vi "test ClearData.vi"(8 "error in (no error)":errorcluster, 11 "TestCase in":refnum<class "Data Manipulation Tests.lvclass">) -> (0 "error out":errorcluster, 3 "TestCase out":refnum<class "Data Manipulation Tests.lvclass">)   [LabVIEW 2017, in "Pointer Tests.lvlib" / "Data Manipulation Tests.lvclass"]
uses:
  Data Manipulation Tests.lvclass
  Source/Classes/Pointer/Public/New/New (1B).vi
  Source/Classes/Pointer/Public/Write/Write (1D U8).vi
  Source/Classes/Pointer/Public/Read/Read (1D U8).vi
  <vilib>/addons/_JKI Toolkits/VI Tester/TestCase.llb/TestCase.lvclass
  Source/Classes/Pointer/Pointer.lvclass
  C:/Program Files (x86)/National Instruments/LabVIEW 2017/vi.lib/addons/_JKI Toolkits/VI Tester/TestCase.llb/TestCase.lvclass
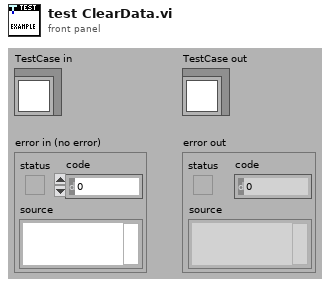
[diagram p1: front panel]
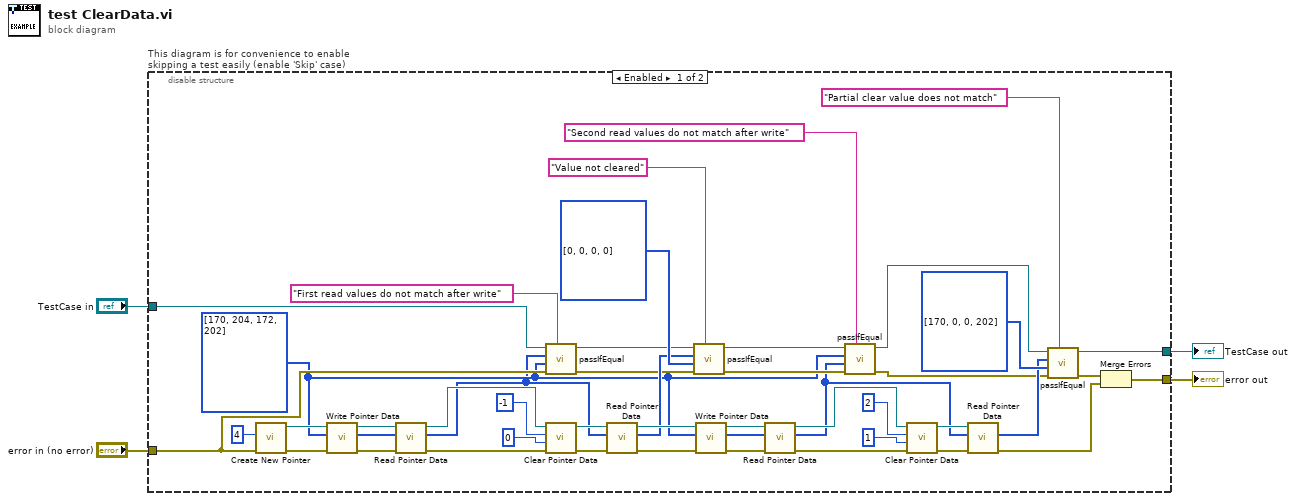
[diagram p0: block diagram]
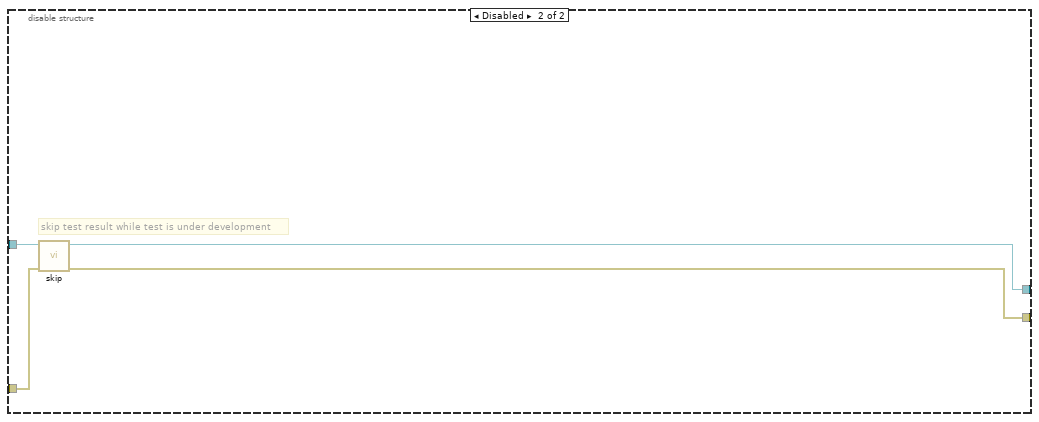
[diagram p2: hidden frame]
diagram:
  n1 = disable-structure "This diagram is for convenience to enable skipping a test easily (enable 'Skip' case)" shown="Enabled" {
    disable-tunnel: "TestCase in" -> [w23 w54]
    disable-tunnel: [w41 w52] -> w1
    disable-tunnel: [w38 w53] -> w3
    disable-tunnel: "error in (no error)" -> [w21 w51]
    frame Enabled {
      w9 = u8[] [170, 204, 172, 202] ("buffer in")
      n2 = call-poly "Create New Pointer.vi"("error in (no error)"=w21, "count (1)"=u64 4) -> ("error out"=w40:errorcluster, "Pointer"=w50:refnum<class "Pointer.lvclass">)  [unwired: 8 in]
      n3 = call-poly "Write Pointer Data.vi"("error in (no error)"=w40, "buffer in"=w9, "Pointer in"=w50) -> ("error out"=w36:errorcluster, "buffer out"=w8:u8[], "Pointer out"=w25:refnum<class "Pointer.lvclass">)  [unwired: 5 in, 1 out]
      n4 = call-poly "Read Pointer Data.vi"("error in (no error)"=w36, "buffer in"=w8, "Pointer in"=w25) -> ("error out"=w26:errorcluster, "buffer out"=w7:u8[], "Pointer out"=w24:refnum<class "Pointer.lvclass">)  [unwired: 5 in, 1 out]
      n5 = call-dynamic "passIfEqual.vi"("custom report message (\"\")"="First read values do not match after write" ("custom report message (\"\")"), "error in (no error)"=w21, "y"=w9, "x"=w7, "TestCase in"=w23) -> ("error out"=w20:errorcluster, "TestCase out"=w22:refnum<class "Data Manipulation Tests.lvclass">)  [unwired: 5 in]
      n6 = call "Clear Pointer Data.vi"("error in (no error)"=w26, "offset (0)"=u64 0, "length (-1: rest)"=i64 -1, "Pointer in"=w24) -> ("error out"=w35:errorcluster, "Pointer out"=w34:refnum<class "Pointer.lvclass">)  [unwired: 6 in]
      n7 = call-poly "Read Pointer Data.vi"("error in (no error)"=w35, "buffer in"=w7, "Pointer in"=w34) -> ("error out"=w39:errorcluster, "buffer out"=w33:u8[], "Pointer out"=w48:refnum<class "Pointer.lvclass">)  [unwired: 5 in, 1 out]
      n8 = call-dynamic "passIfEqual.vi"("custom report message (\"\")"="Value not cleared" ("custom report message (\"\")"), "error in (no error)"=w20, "y"=u8[] [0, 0, 0, 0] ("buffer in"), "x"=w33, "TestCase in"=w22) -> ("error out"=w43:errorcluster, "TestCase out"=w15:refnum<class "Data Manipulation Tests.lvclass">)  [unwired: 5 in]
      n9 = call-poly "Write Pointer Data.vi"("error in (no error)"=w39, "buffer in"=w9, "Pointer in"=w48) -> ("error out"=w47:errorcluster, "buffer out"=w6:u8[], "Pointer out"=w18:refnum<class "Pointer.lvclass">)  [unwired: 5 in, 1 out]
      n10 = call-poly "Read Pointer Data.vi"("error in (no error)"=w47, "buffer in"=w6, "Pointer in"=w18) -> ("error out"=w19:errorcluster, "buffer out"=w5:u8[], "Pointer out"=w17:refnum<class "Pointer.lvclass">)  [unwired: 5 in, 1 out]
      n11 = call-dynamic "passIfEqual.vi"("custom report message (\"\")"="Second read values do not match after write" ("custom report message (\"\")"), "error in (no error)"=w43, "y"=w5, "x"=w9, "TestCase in"=w15) -> ("error out"=w16:errorcluster, "TestCase out"=w14:refnum<class "Data Manipulation Tests.lvclass">)  [unwired: 5 in]
      n12 = call "Clear Pointer Data.vi"("error in (no error)"=w19, "offset (0)"=u64 1, "length (-1: rest)"=i64 2, "Pointer in"=w17) -> ("error out"=w32:errorcluster, "Pointer out"=w31:refnum<class "Pointer.lvclass">)  [unwired: 6 in]
      n13 = call-poly "Read Pointer Data.vi"("error in (no error)"=w32, "buffer in"=w5, "Pointer in"=w31) -> ("error out"=w37:errorcluster, "buffer out"=w44:u8[])  [unwired: 5 in, 2 out]
      n14 = call-dynamic "passIfEqual.vi"("custom report message (\"\")"="Partial clear value does not match" ("custom report message (\"\")"), "error in (no error)"=w16, "y"=u8[] [170, 0, 0, 202] ("buffer in"), "x"=w44, "TestCase in"=w14) -> ("error out"=w42:errorcluster, "TestCase out"=w41:refnum<class "Data Manipulation Tests.lvclass">)  [unwired: 5 in]
      n15 = Merge Errors(w42, w37) -> (w38:errorcluster)
    }
    frame Disabled {
      # "skip test result while test is under development"
      n16 = call <vilib>:"skip.vi"("error in (no error)"=w51, "TestCase in"=w54) -> ("error out"=w53:errorcluster, "TestCase out"=w52:refnum<class "Data Manipulation Tests.lvclass">)  [unwired: 8 in]
    }
  }
  "error out" <- w3
  "TestCase out" <- w1
